vi "写入内置参数.vi"(7 "量程参数读取":T3 {"阈值（高->低）" format="%#.6g"; "阈值（低->高）" format="%#.6g"; "下限" format="%#.6g"; "上限" format="%#.6g"}, 8 "error in (no error)":errorcluster, 9 "float":T2 {"偏心轮校准参数" format="%#.6g"}, 10 "外设配置":T1 {"是否存在液位检测板" items=["否", "是"]; "阀数量" items=["9通"=9, "12通"=12]; "泵类型" items=["TECAN", "润泽"]}, 11 "MB session in":refnum<class "MB_Master.lvclass">) -> (0 "error out":errorcluster, 3 "MB session out":refnum<class "MB_Master.lvclass">)   [LabVIEW 2016, in "斯坦道CODMn新电路板.lvlib"]
uses:
  <vilib>/Plasmionique/MB Master/MB_Master/MB_Master.lvclass
  <vilib>/Plasmionique/MB Master/MB_Master_Serial/MB_Master_Serial.lvclass
  C:/Program Files (x86)/National Instruments/LabVIEW 2016/vi.lib/Plasmionique/MB Master/MB_Master/MB_Master.lvclass
  <vilib>/Plasmionique/MB Master/MB Master.lvlib
panel:
  in  "VISA Resource":refnum<visa-resource-name>
  in  "引用选择":enum16{"MB引用", "自建引用"}(ring)
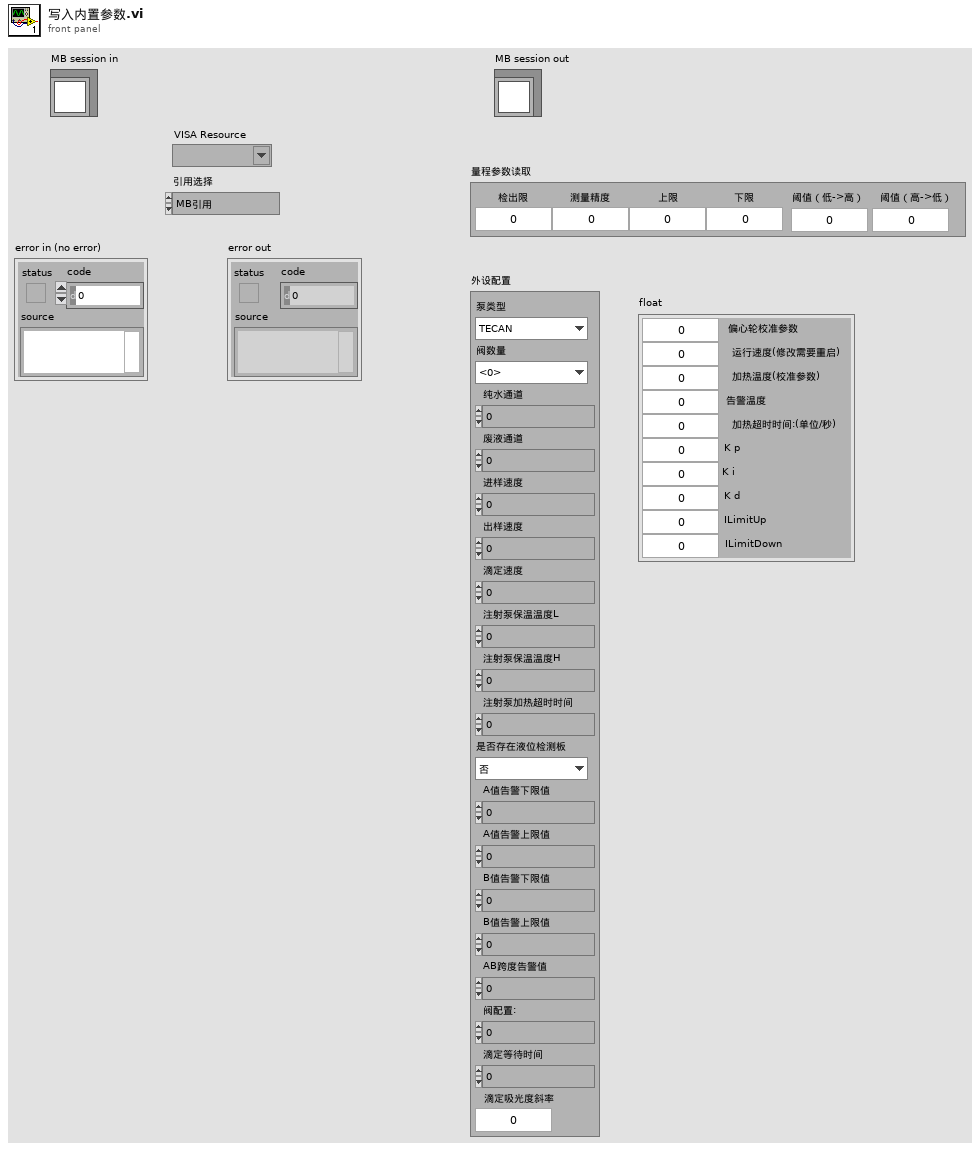
[diagram p1: front panel]
types:
  T1 = cluster{"泵类型":u8, "阀数量":u8, "纯水通道":u8, "废液通道":u8, "进样速度":u16, "出样速度":u16, "滴定速度":u16, "注射泵保温温度L":u8, "注射泵保温温度H":u8, "注射泵加热超时时间":u16, "是否存在液位检测板":u16, "A值告警下限值":u16, "A值告警上限值":u16, "B值告警下限值":u16, "B值告警上限值":u16, "AB跨度告警值":u16, "阀配置:":u8, "滴定等待时间":u16, "滴定吸光度斜率":dbl}
  T2 = cluster{"偏心轮校准参数":dbl, "运行速度(修改需要重启)":u16, "加热温度(校准参数) ":dbl, "告警温度":dbl, "加热超时时间:(单位/秒)":dbl, "K p":dbl, "K i":dbl, "K d":dbl, "ILimitUp":dbl, "ILimitDown":dbl}
  T3 = cluster{"检出限":dbl, "测量精度":dbl, "上限":dbl, "下限":dbl, "阈值（低->高）":dbl, "阈值（高->低）":dbl}
  T4 = cluster{"baud rate (bps)":u32, "stop bits":u16, "parity":u16, "flow control":u16, "timeout":u32, "retries":i32}
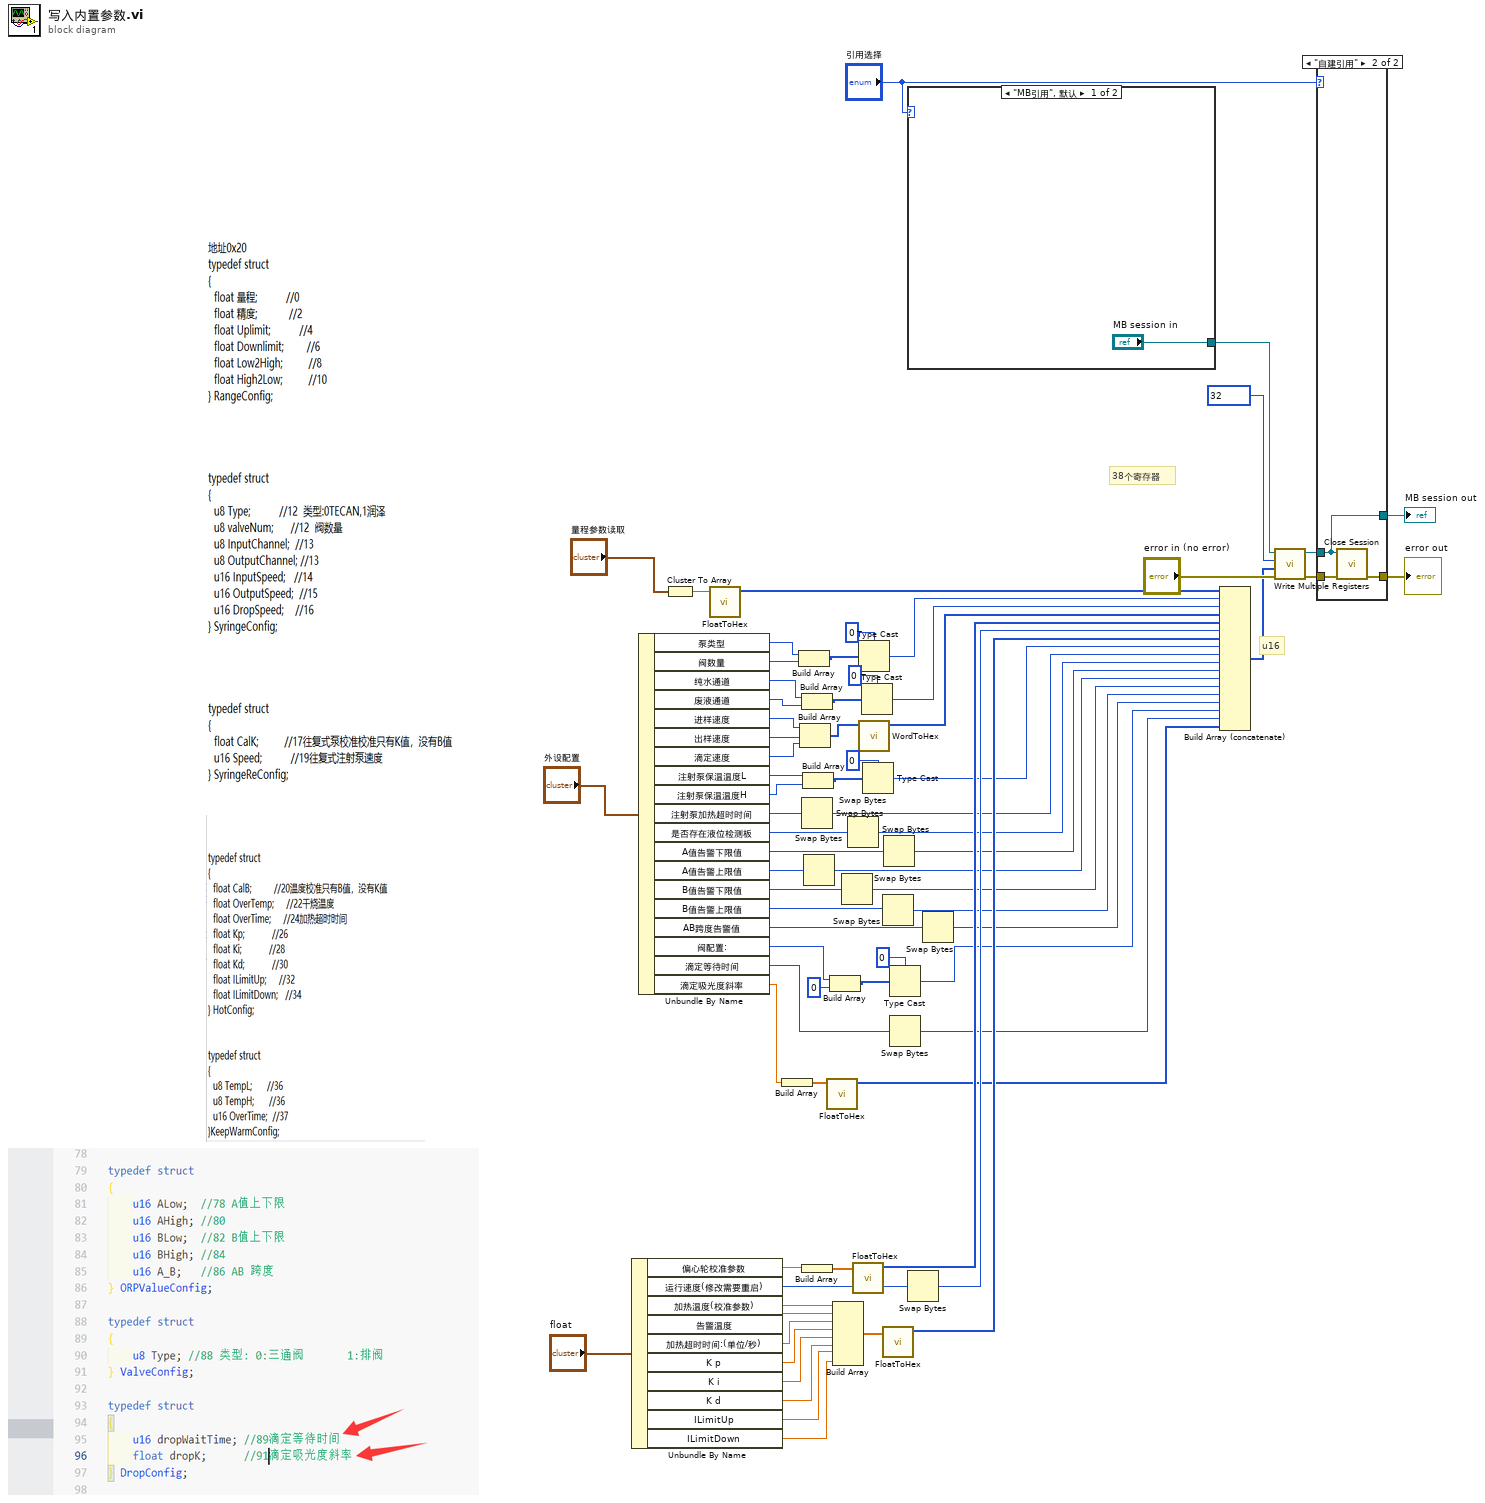
[diagram p0: block diagram]
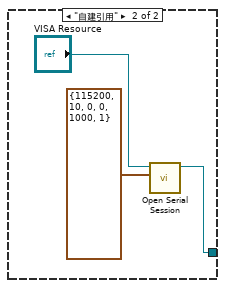
[diagram p3: hidden frame]
diagram:
  # "38个寄存器"
  # "u16"
  n1 = Unbundle By Name("float") -> ("偏心轮校准参数"=w51:dbl, "运行速度(修改需要重启)"=w28:u16, "加热温度(校准参数)"=w48:dbl, "告警温度"=w47:dbl, "加热超时时间:(单位/秒)"=w46:dbl, "K p"=w45:dbl, "K i"=w44:dbl, "K d"=w43:dbl, "ILimitUp"=w42:dbl, "ILimitDown"=w41:dbl)
  n2 = Unbundle By Name("外设配置") -> ("泵类型"=w63:u8, "阀数量"=w62:u8, "纯水通道"=w56:u8, "废液通道"=w55:u8, "进样速度"=w34:u16, "出样速度"=w33:u16, "滴定速度"=w32:u16, "注射泵保温温度L"=w37:u8, "注射泵保温温度H"=w36:u8, "注射泵加热超时时间"=w35:u16, "是否存在液位检测板"=w23:u16, "A值告警下限值"=w21:u16, "A值告警上限值"=w20:u16, "B值告警下限值"=w19:u16, "B值告警上限值"=w18:u16, "AB跨度告警值"=w17:u16, "阀配置:"=w9:u8, "滴定等待时间"=w6:u16, "滴定吸光度斜率"=w4:dbl)
  n3 = Cluster To Array(cluster="量程参数读取") -> (array=w65:dbl[])
  n4 = call "FloatToHex.vi"("浮点数"=w65) -> ("DCBA整形输出"=w64:u16[])  [unwired: 10 in]
  n5 = Build Array(w4) -> (w3:dbl[])
  n6 = Build Array(w63, w62) -> (w59:u8[])
  n7 = Build Array(w34, w33, w32) -> (w31:u16[])
  n8 = Build Array(w56, w55) -> (w58:u8[])
  n9 = Swap Bytes(anything=w35) -> (byte swapped=w24:u16)
  n10 = Build Array(w51) -> (w50:dbl[])
  n11 = Build Array(w37, w36) -> (w39:u8[])
  n12 = Swap Bytes(anything=w20) -> (byte swapped=w15:u16)
  n13 = call "FloatToHex.vi"("浮点数"=w3) -> ("DCBA整形输出"=w2:u16[])  [unwired: 10 in]
  n14 = Build Array(w9, u8 0 ("元素")) -> (w10:u8[])
  n15 = Build Array(w48, w47, w46, w45, w44, w43, w42, w41) -> (w40:dbl[])
  n16 = Swap Bytes(anything=w19) -> (byte swapped=w14:u16)
  n17 = Swap Bytes(anything=w23) -> (byte swapped=w22:u16)
  n18 = call "FloatToHex.vi"("浮点数"=w50) -> ("DCBA整形输出"=w29:u16[])  [unwired: 10 in]
  n19 = Type Cast(type=u16 0, x=w59) -> (*(type *) &x=w53:u16)
  n20 = call "WordToHex.vi"("WORD"=w31) -> ("数组"=w30:u16[])  [unwired: 10 in]
  n21 = Type Cast(type=u16 0, x=w58) -> (*(type *) &x=w52:u16)
  n22 = Type Cast(type=u16 0, x=w39) -> (*(type *) &x=w25:u16)
  n23 = Swap Bytes(anything=w18) -> (byte swapped=w13:u16)
  n24 = call "FloatToHex.vi"("浮点数"=w40) -> ("DCBA整形输出"=w26:u16[])  [unwired: 10 in]
  n25 = Swap Bytes(anything=w21) -> (byte swapped=w16:u16)
  n26 = Type Cast(type=u16 0, x=w10) -> (*(type *) &x=w8:u16)
  n27 = Swap Bytes(anything=w6) -> (byte swapped=w5:u16)
  n28 = case shown="\"MB引用\", 默认" "引用选择" {
    tunnel: ["MB session in" w77] -> w71
    frame "MB引用", Default {
    }
    frame "自建引用" {
      n29 = call <vilib>:"Open Serial Session.vi"("Serial Config"=T4 {"baud rate (bps)"=115200, "stop bits"=10, "parity"=0, "flow control"=0, "timeout"=1000, "retries"=1}, "VISA Resource"="VISA Resource") -> ("MB_Serial session"=w77:refnum<class "MB_Master_Serial.lvclass">)  [unwired: 8 in, 1 out]
    }
  }
  n30 = Swap Bytes(anything=w28) -> (byte swapped=w27:u16)
  n31 = Swap Bytes(anything=w17) -> (byte swapped=w12:u16)
  n32 = Build Array (concatenate)(w64, w53, w52, w30, w29, w27, w26, w25, w24, w22, w16, w15, w14, w13, w12, w8, w5, w2) -> (w54:u16[])
  n33 = call <vilib>:"Write Multiple Registers.vi"("error in (no error)"="error in (no error)", "values"=w54, "starting address"=u16 32, "MB session in"=w71) -> ("error out"=w68:errorcluster, "MB session out"=w70:refnum<class "MB_Master.lvclass">)  [unwired: 6 in]
  n34 = case shown="\"自建引用\"" "引用选择" {
    tunnel: w70 -> [w78 w80]
    tunnel: w68 -> [w79 w82]
    tunnel: [w79 w81] -> w67
    tunnel: [w78 w80] -> w66
    frame "MB引用", Default {
    }
    frame "自建引用" {
      n35 = call-dynamic "Close Session.vi"("error in (no error)"=w82, "MB session in"=w80) -> ("error out"=w81:errorcluster)  [unwired: 9 in]
    }
  }
  "MB session out" <- w66
  "error out" <- w67
